vi "Display Frame Rate Control (SubVI).vi"(6 "Pixel Valid":bool, 8 "Image Width":u16, 10 "Image Height":u16, 12 "Frame Int.":u16) -> (14 "Enable":bool, 19 "EOF?":bool)   [LabVIEW 2015]
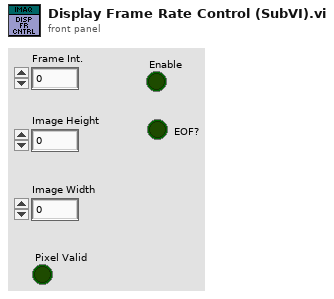
[diagram p1: front panel]
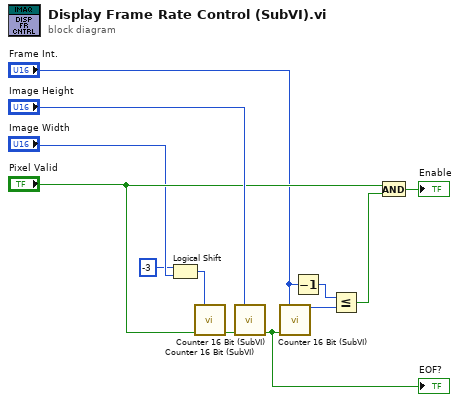
[diagram p0: block diagram]
diagram:
  n1 = Logical Shift(y=i16 -3, x="Image Width") -> (x << y=w4:u16)
  n2 = call "Counter 16 Bit (SubVI).vi"("Max. Count"=w4, "Enable"="Pixel Valid") -> ("Count End?"=w3:bool)  [unwired: 11 in, 2 out]
  n3 = call "Counter 16 Bit (SubVI).vi"("Max. Count"="Image Height", "Enable"=w3) -> ("Count End?"=w9:bool)  [unwired: 11 in, 2 out]
  "EOF?" <- w9
  n4 = call "Counter 16 Bit (SubVI).vi"("Max. Count"="Frame Int.", "Enable"=w9) -> ("Count"=w10:u16)  [unwired: 11 in, 2 out]
  n5 = Decrement(x="Frame Int.") -> (x-1=w1:u16)
  n6 = Less Or Equal?(x=w1, y=w10) -> (x <= y?=w12:bool)
  n7 = And(x="Pixel Valid", y=w12) -> (x .and. y?=→"Enable":bool)
